vi "Event Handler.vi"(8 "error in (no error)":errorcluster, 10 "Stop Event Handler":refnum<user-event>, 11 "SwipeScrollListbox in":refnum<class "SwipeScrollListbox.lvclass">) -> (0 "error out":errorcluster)   [LabVIEW 2019, in "SwipeScrollListbox.lvclass"]
doc: "The <b>Event Handler VI</b> is a dynamic dispatch VI that should be overwritten if events are needed to create the enhanced QControl. \n\nBy inheriting from the main Control.lvclass the overwritten <b>Event Handler VI</b> will be launched asynchronously in the initialization of the QControl.\n<b> </b> <b> </b>\n©2016 Q Software Innovations, LLC (QSI)\nwritten by Quentin Alldredge\nproduced in LabVIEW 2015\n\nsupport@qsoftwareinnovations.com\nwww.qsoftwareinnovations.com\n\nAll rights reserved.\n\nRedistribution and use in source and binary forms, with or without modification, are permitted provided that the following conditions are met:\n\n * Redistributions of source code must retain the above copyright notice, this list of conditions and the following disclaimer.\n * Redistributions in binary form must reproduce the above copyright notice, this list of conditions and the following disclaimer in the documentation and/or other materials provided with the distribution.\n * Neither the name of Q Software Innovations, LLC. nor the names of its contributors may be used to endorse or promote products derived from this software without specific prior written permission.\n\nTHIS SOFTWARE IS PROVIDED BY THE COPYRIGHT HOLDERS AND CONTRIBUTORS \"AS IS\" AND ANY EXPRESS OR IMPLIED WARRANTIES, INCLUDING, BUT NOT LIMITED TO, THE IMPLIED WARRANTIES OF MERCHANTABILITY AND FITNESS FOR A PARTICULAR PURPOSE ARE DISCLAIMED. IN NO EVENT SHALL THE COPYRIGHT OWNER OR CONTRIBUTORS BE LIABLE FOR ANY DIRECT, INDIRECT, INCIDENTAL, SPECIAL, EXEMPLARY, OR CONSEQUENTIAL DAMAGES (INCLUDING, BUT NOT LIMITED TO, PROCUREMENT OF SUBSTITUTE GOODS OR SERVICES; LOSS OF USE, DATA, OR PROFITS; OR BUSINESS INTERRUPTION) HOWEVER CAUSED AND ON ANY THEORY OF LIABILITY, WHETHER IN CONTRACT, STRICT LIABILITY, OR TORT (INCLUDING NEGLIGENCE OR OTHERWISE) ARISING IN ANY WAY OUT OF THE USE OF THIS SOFTWARE, EVEN IF ADVISED OF THE POSSIBILITY OF SUCH DAMAGE."
uses:
  SwipeScrollListbox.lvclass
  SwipeScrollListbox.lvclass/SwipeScrollListbox.ctl
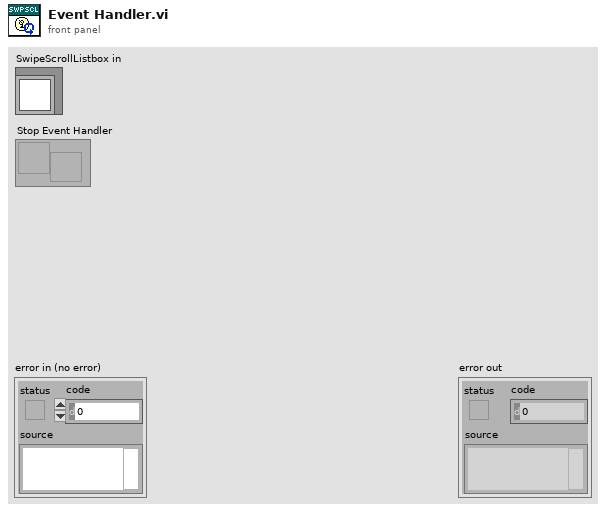
[diagram p1: front panel]
types:
  T1 = typedef "LVPoint32TypeDef.ctl" = cluster{"Horizontal":i32, "Vertical":i32}
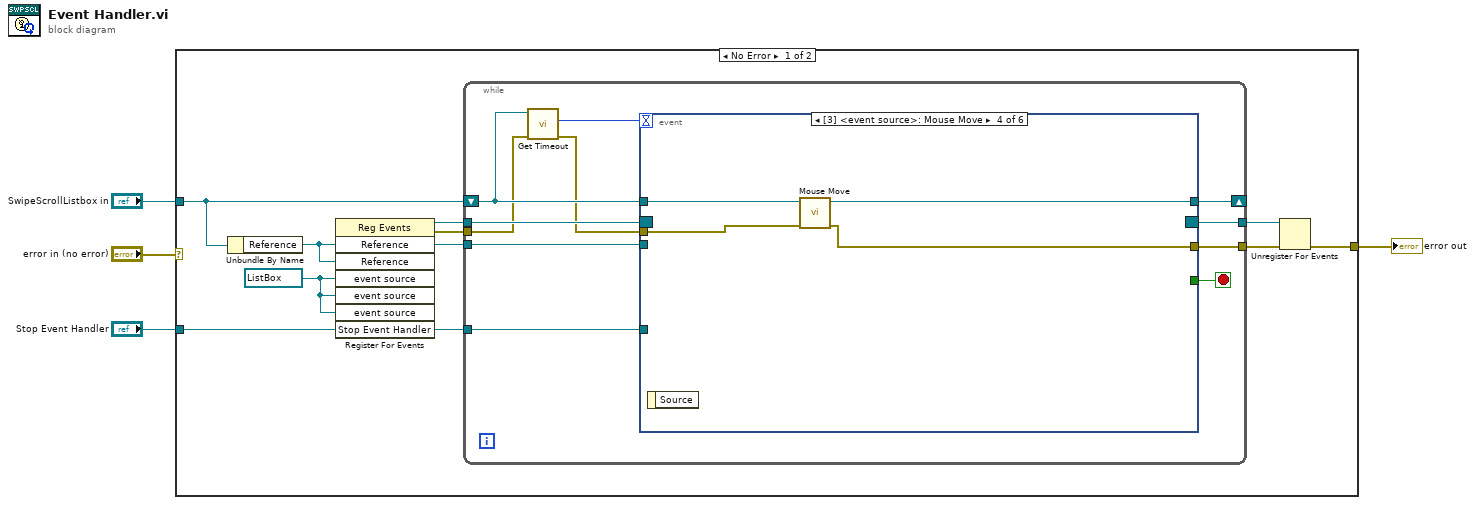
[diagram p0: block diagram]
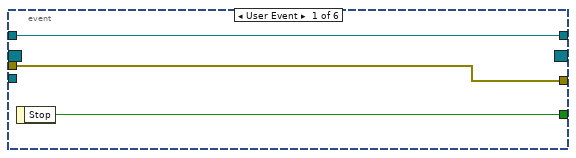
[diagram p2: hidden frame]
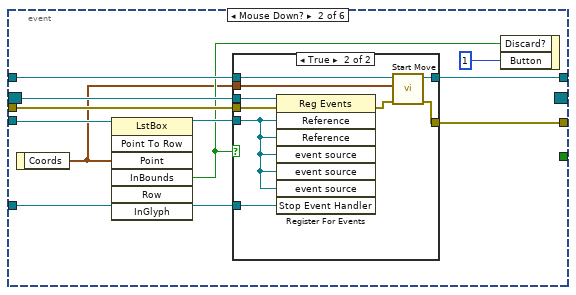
[diagram p3: hidden frame]
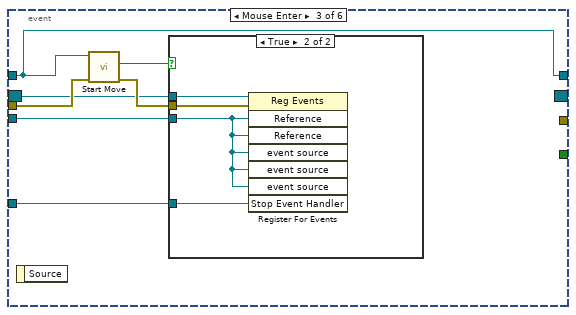
[diagram p5: hidden frame]
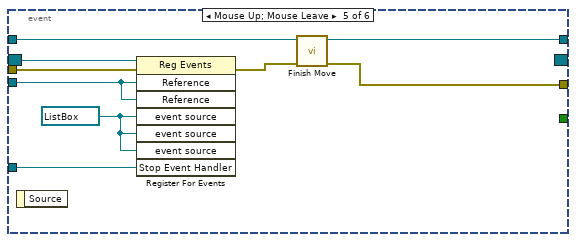
[diagram p7: hidden frame]
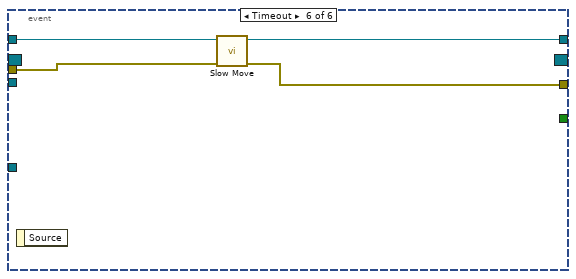
[diagram p8: hidden frame]
diagram:
  n1 = case shown="No Error" "error in (no error)" {
    selector: "error in (no error)" -> [_ w78]
    tunnel: [w10 w78] -> w3
    tunnel: "SwipeScrollListbox in" -> [w8 _]
    tunnel: "Stop Event Handler" -> [w6 _]
    frame No Error {
      w5 = refnum<vi> refnum ("event source")
      n2 = Unbundle By Name(w8) -> ("Reference"=w7:refnum<vi>)
      n3 = register-events(w7, w7, w5, w5, w5, w6) -> (reference out=w13:refnum<event-registration>, error out=w12:errorcluster)  [unwired: 2 in]
      n4 = while {
        tunnel: w13 -> [w24]
        tunnel: w12 -> [w14]
        tunnel: [w23] -> w11
        tunnel: [w21] -> w9
        tunnel: w7 -> [w20]
        tunnel: w6 -> [w19]
        shift-right: [w18] -> _
        shift-left: w8 -> [w17]
        stop <- w22 stop-if-true
        n5 = call "Get Timeout.vi"("error in (no error)"=w14, "SwipeScrollListbox in"=w17) -> ("error out"=w15:errorcluster, "Timeout"=w16:i32)  [unwired: 7 in, 1 out]
        n6 = event shown="[3] <event source>: Mouse Move" {
          selector: w24 -> [_ w35 w51 _ w71 _]
          dyn-events: [_ _ _ _ _ _] -> w21
          timeout: w16 -> [_ _ _ _ _ _]
          tunnel: w17 -> [w25 w36 w54 w63 w69 w77]
          tunnel: w15 -> [w27 w37 w53 w62 w72 w75]
          tunnel: [w27 w29 _ w61 w67 w74] -> w23
          tunnel: [w26 _ _ _ _ _] -> w22
          tunnel: w20 -> [_ w32 w55 _ w73 _]
          tunnel: w19 -> [_ w38 w56 _ w65 _]
          tunnel: [w25 w33 w54 w64 w70 w76] -> w18
          event User Event {
            n7 = event-data() -> ("Stop"=w26:bool)  [unwired: 1 in]
          }
          event Mouse Down? {
            n8 = event-data() -> ("Coords"=w28:T1)  [unwired: 1 in]
            n9 = invoke class="LstBox" method="Point To Row"(reference=w32, "Point"=w28) -> (reference out=w31:refnum<vi>, "InBounds"=w30:bool)  [unwired: 5 in, 5 out]
            n10 = case shown="True" w30 {
              tunnel: w38 -> [_ w49]
              tunnel: w37 -> [w39 w48]
              tunnel: w36 -> [w40 w47]
              tunnel: w35 -> [_ w46]
              tunnel: [w40 w45] -> w33
              tunnel: w31 -> [_ w44]
              tunnel: [w39 w42] -> w29
              tunnel: w28 -> [_ w41]
              frame False {
              }
              frame True {
                n11 = register-events(reference=w46, error in=w48, w44, w44, w44, w44, w44, w49) -> (error out=w43:errorcluster)  [unwired: 1 out]
                n12 = call "Start Move.vi"("error in (no error)"=w43, "Coords"=w41, "SwipeScrollListbox in"=w47) -> ("error out"=w42:errorcluster, "SwipeScrollListbox out"=w45:refnum<class "SwipeScrollListbox.lvclass">)  [unwired: 6 in, 1 out]
              }
            }
            n13 = event-data("Discard?"=w30, "Button"=u16 1) -> ()  [unwired: 1 in, 1 out]
          }
          event Mouse Enter {
            n14 = event-data() -> ()  [unwired: 1 in, 1 out]
            n15 = call "Start Move.vi"("error in (no error)"=w53, "SwipeScrollListbox in"=w54) -> ("error out"=w52:errorcluster, "Button Down"=w50:bool)  [unwired: 7 in, 1 out]
            n16 = case shown="True" w50 {
              tunnel: w56 -> [_ w60]
              tunnel: w55 -> [_ w59]
              tunnel: w52 -> [_ w58]
              tunnel: w51 -> [_ w57]
              frame False {
              }
              frame True {
                n17 = register-events(reference=w57, error in=w58, w59, w59, w59, w59, w59, w60) -> ()  [unwired: 2 out]
              }
            }
          }
          event Mouse Move {
            n18 = event-data() -> ()  [unwired: 1 in, 1 out]
            n19 = call "Mouse Move.vi"("error in (no error)"=w62, "SwipeScrollListbox in"=w63) -> ("error out"=w61:errorcluster, "SwipeScrollListbox out"=w64:refnum<class "SwipeScrollListbox.lvclass">)  [unwired: 8 in]
          }
          event Mouse Up; Mouse Leave {
            w66 = refnum<vi> refnum ("event source")
            n20 = event-data() -> ()  [unwired: 1 in, 1 out]
            n21 = register-events(reference=w71, error in=w72, w73, w73, w66, w66, w66, w65) -> (error out=w68:errorcluster)  [unwired: 1 out]
            n22 = call "Finish Move.vi"("error in (no error)"=w68, "SwipeScrollListbox in"=w69) -> ("error out"=w67:errorcluster, "SwipeScrollListbox out"=w70:refnum<class "SwipeScrollListbox.lvclass">)  [unwired: 8 in]
          }
          event Timeout {
            n23 = event-data() -> ()  [unwired: 1 in, 1 out]
            n24 = call "Slow Move.vi"("error in (no error)"=w75, "SwipeScrollListbox in"=w77) -> ("error out"=w74:errorcluster, "SwipeScrollListbox out"=w76:refnum<class "SwipeScrollListbox.lvclass">)  [unwired: 8 in]
          }
        }
      }
      n25 = Unregister For Events(event registration refnum=w9, error in=w11) -> (error out=w10:errorcluster)
    }
    frame Error {
    }
  }
  "error out" <- w3
